vi "Run SerDes Config Scripts.vi"(6 "Complex Serdes Scripts":bool, 8 "error in (no error)":errorcluster, 9 "configuration scripts":path, 10 "serial channels":string, 11 "FPGA Ref In":refnum<k20>) -> (0 "error out":errorcluster, 2 "script output":string[](array[string]), 3 "FPGA Ref Out":refnum<k20>)   [LabVIEW 2025, in "I2C Bus Monitor.lvclass"]
uses:
  I2C Bus Monitor.lvclass
  I2C Bus Monitor.lvclass/I2C Bus Monitor.ctl
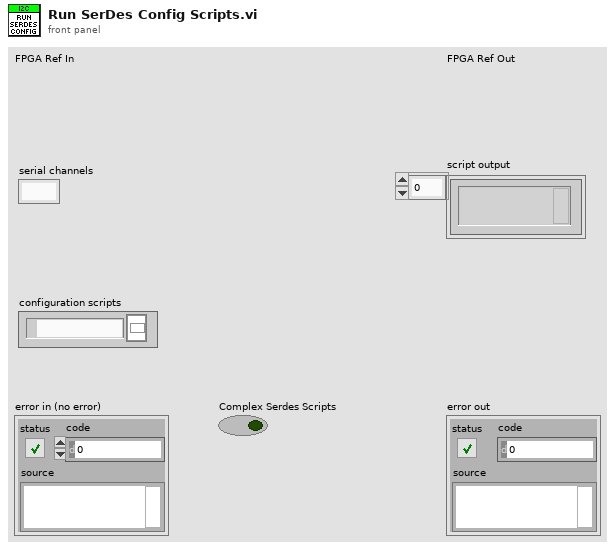
[diagram p1: front panel]
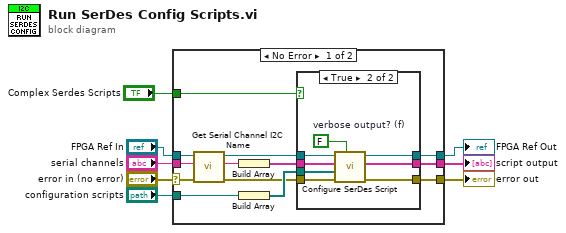
[diagram p0: block diagram]
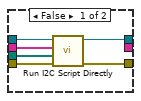
[diagram p2: hidden frame]
diagram:
  n1 = case shown="No Error" "error in (no error)" {
    selector: "error in (no error)" -> [w15 w37]
    tunnel: [w21 _] -> w8
    tunnel: "configuration scripts" -> [w20 _]
    tunnel: "serial channels" -> [w11 _]
    tunnel: [w19 w37] -> w4
    tunnel: "FPGA Ref In" -> [w14 w36]
    tunnel: [w18 w36] -> w2
    tunnel: "Complex Serdes Scripts" -> [w17 _]
    frame No Error {
      n2 = call "Get Serial Channel I2C Name.vi"("error in (no error)"=w15, "Serial Channel"=w11, "FGPA Ref in"=w14) -> ("error out"=w12:errorcluster, "SO/SI I2C Name"=w10:string, "FPGA Ref out"=w13:refnum<k20>)  [unwired: 6 in]
      n3 = Build Array(w10) -> (w9:string[])
      n4 = Build Array(w20) -> (w16:path[])
      n5 = case shown="True" w17 {
        tunnel: [_ w35] -> w21
        tunnel: w16 -> [w26 w34]
        tunnel: [w22 w33] -> w19
        tunnel: w13 -> [w24 w32]
        tunnel: [w23 w31] -> w18
        tunnel: w12 -> [w27 w30]
        tunnel: w9 -> [w25 w28]
        frame False {
          n6 = call "Run I2C Script Directly.vi"("error in"=w27, "configuration scripts"=w26, "serial channels"=w25, "FPGA Ref In"=w24) -> ("error out"=w22:errorcluster, "FPGA Ref Out"=w23:refnum<k20>)  [unwired: 6 in]
        }
        frame True {
          w29 = FALSE  # verbose output? (f)
          n7 = call "Configure SerDes Script.vi"("verbose? (T)"=w29, "error in"=w30, "scripts"=w34, "bus instance names"=w28, "FPGA Ref In"=w32) -> ("error out"=w33:errorcluster, "outputs"=w35:string[], "FPGA Ref Out"=w31:refnum<k20>)  [unwired: 4 in]
        }
      }
    }
    frame Error {
    }
  }
  "script output" <- w8
  "FPGA Ref Out" <- w2
  "error out" <- w4
